vi "CovertToStringSubVi.vi"(1 "input":dbl) -> (0 "resulting string":string)   [LabVIEW 2015]
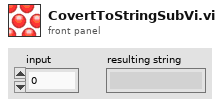
[diagram p1: front panel]
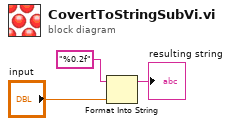
[diagram p0: block diagram]
diagram:
  n1 = Format Into String(format string="%0.2f", "input") -> (resulting string=→"resulting string":string)  [unwired: 2 in, 1 out]
